vi "PID Percentage to EGU (DBL Array).vi"(1 "coerce output to range? (T)":bool=TRUE, 2 "minimum (EGU)":dbl[](array[numeric])=[0.0] format="%.2f", 3 "% span":dbl[](array[numeric])=[0.0] format="%.2f", 4 "maximum (EGU)":dbl[](array[numeric])=[0.0] format="%.2f") -> (0 "output (EGU)":dbl[](array[numeric]) format="%.2f")   [LabVIEW 2017, in "NI_PID_pid.lvlib"]
doc: "Converts a percent-of-range input to an engineering-units output based on the minimum and maximum range settings. The output is normally limited to the range [max...min]. Values outside of the range [max..min] are allowed when <B>coerce output to range?</B> is FALSE. Use the DBL instance of this VI to implement a single control loop. Use the DBL Array instance to implement parallel multi-loop control."
uses:
  <vilib>/addons/control/pid/NI_PID_pid.lvlib
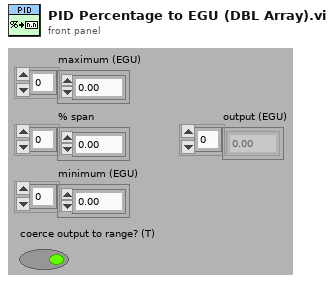
[diagram p1: front panel]
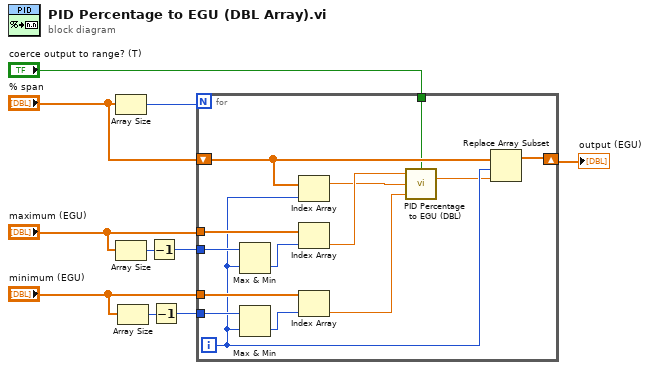
[diagram p0: block diagram]
diagram:
  n1 = Array Size(array="% span") -> (size(s)=w6:i32)
  n2 = Array Size(array="maximum (EGU)") -> (size(s)=w10:i32)
  n3 = Array Size(array="minimum (EGU)") -> (size(s)=w8:i32)
  n4 = Decrement(x=w10) -> (x-1=w9:i32)
  n5 = Decrement(x=w8) -> (x-1=w7:i32)
  n6 = for {
    N: w6 -> [_]
    tunnel: "maximum (EGU)" -> [w21]
    tunnel: "minimum (EGU)" -> [w22]
    shift-right: [w23] -> w2
    shift-left: "% span" -> [w24]
    tunnel: w9 -> [w20]
    tunnel: w7 -> [w19]
    tunnel: "coerce output to range? (T)" -> [w11]
    i -> [w16]
    n7 = Max & Min(x=w20, y=w16) -> (min(x,y)=w17:i32)  [unwired: 1 out]
    n8 = Max & Min(x=w19, y=w16) -> (min(x,y)=w18:i32)  [unwired: 1 out]
    n9 = Index Array(array=w24, index=w16) -> (element=w14:dbl)
    n10 = Index Array(array=w21, index=w17) -> (element=w15:dbl)
    n11 = Index Array(array=w22, index=w18) -> (element=w13:dbl)
    n12 = call <vilib>:"PID Percentage to EGU (DBL).vi"("coerce output to range? (T)"=w11, "minimum (EGU)"=w13, "% span"=w14, "maximum (EGU)"=w15) -> ("output (EGU)"=w12:dbl)
    n13 = Replace Array Subset(array=w24, new element=w12, index=w16) -> (w23:dbl[])
  }
  "output (EGU)" <- w2
